vi "Set Test Timestamp.vi"(8 "error in (no error)":errorcluster, 10 "Test Timestamp":timestamp, 11 "Submission in":refnum<class "Submission.lvclass">) -> (0 "error out":errorcluster, 3 "Submission out":refnum<class "Submission.lvclass">)   [LabVIEW 2020, in "Summer of LabVIEW.lvlib" / "Submission.lvclass"]
uses:
  Submission.lvclass
  Submission.lvclass/Submission.ctl
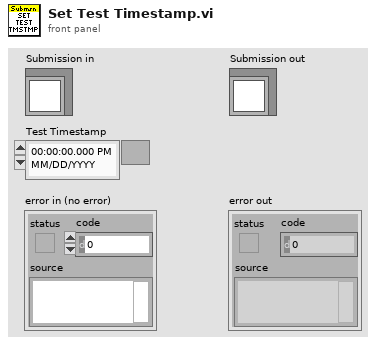
[diagram p1: front panel]
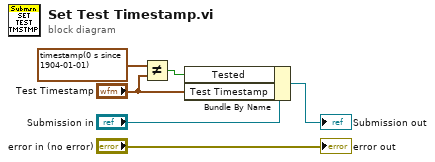
[diagram p0: block diagram]
diagram:
  n1 = Not Equal?(x=timestamp(0 s since 1904-01-01) ("Test Timestamp"), y="Test Timestamp") -> (x != y?=w1:bool)
  n2 = Bundle By Name(cluster="Submission in", "Tested"=w1, "Test Timestamp"="Test Timestamp") -> (→"Submission out":refnum<class "Submission.lvclass">)
  "error out" <- "error in (no error)"
